vi "Receive - UDP (CommPort).vi"() -> ()   [LabVIEW 2020]
uses:
  <instrlib>/AIM GmbH/_AIM 664/_controls/comm_verification_rx.ctl
  <instrlib>/AIM GmbH/_AIM 664/_controls/comm_udp_rx.ctl
  <instrlib>/AIM GmbH/_AIM 664/_polimorphicInstances/session/CreateSession(Rx-VL-Oriented).vi
  <instrlib>/AIM GmbH/_AIM 664/bsp/AFDX_Receive/Create Rx VL.vi
  <instrlib>/AIM GmbH/_AIM 664/_polimorphicInstances/udpPort/CreateUdpPort(RX-CommPort).vi
  <instrlib>/AIM GmbH/_AIM 664/_polimorphicInstances/control/Start (Rx).vi
  <instrlib>/AIM GmbH/_AIM 664/_polimorphicInstances/control/Stop (Rx).vi
  <instrlib>/AIM GmbH/_AIM 664/_polimorphicInstances/session/CleanupSession (Port).vi
  <instrlib>/AIM GmbH/_AIM 664/AIM664LV.lvlib
panel:
  out "Curent Irig Time":T1
  in  "CommPort Config":T2={"PortType"=enum."FDX_UDP_SAMPLING", "SubVIId"=1, "domainID"=1, "sideID"=1, "locationID"=1, "partitionID"=1, "UdpSrcPort"=12345, "UdpDstPort"=12346, "UdpNumBufMessages"=0, "UdpMaxMessageSize"=1000, "UdpSamplingRate"=0} {"partitionID" format="%.0b"}
  out "BytesRead":u32
  out "Data":u8[](array[numeric])=[1, 2, 3, 4, 0, 0, 0, 0, 0, 0, 0, 0, 0, 0, 0, 0, 0, 0, 0, 0, 0, 0, 0, 0, 0, 0, 0, 0, 0, 0, 0, 0, 0, 0, 0, 0, 0, 0, 0, 0, 0, 0, 0, 0, 0, 0, 0, 0, 0, 0, 0, 0, 0, 0, 0, 0, 0, 0, 0, 0, 0, 0, 0, 0, 0, 0, 0, 0, 0, 0, 0, 0, 0, 0, 0, 0, 0, 0, 0, 0, 0, 0, 0, 0, 0, 0, 0, 0, 0, 0, 0, 0, 0, 0, 0, 0, 0, 0, 0, 0] format="%.0x"
  in  "Messages to Read (1)":u32=1
  in  "VL Config":T3={"VlId"=60, "VLRange"=1, "VerificationMode"=0, "Bag"=0, "Jitter"=0, "MaxFrameLength"=0, "MaxSkew"=0, "VLBufSize"=32768, "FilterMode"=0, "FilterPosition"=0, "Padding"=0, "FilterMask"=0, "FilterData"=0, "MinFrameLength"=0} {"FilterMode" items=["FDX_RX_VL_FLT_DIS", "FDX_RX_VL_FLT_ENA ", "FDX_RX_VL_FLT_ENA_INV"]; "MaxFrameLength" format="%.0x"; "VerificationMode" items=["FDX_RX_VL_CHECK_ENA_DEFAULT"=65535, "FDX_RX_VL_CHECK_REDMAM"=16, "DX_RX_VL_CHECK_TRAFIC"=8, "FDX_RX_VL_CHECK_FRAMESIZE"=4, "FDX_RX_VL_CHECK_SNINTEG"=2, "FDX_RX_VL_CHECK_INVPAC"=1, "FDX_RX_VL_CHECK_DISA"=0]}
  out "PortInitOut":T4 {"PortConfig" items=["FDX_SINGLE", "FDX_REDUNDANT"]}
  in  "port":u32=1
  in  "board":u32
  in  "Period mS":u32=200
  out "error out":errorcluster
  in  "stop":bool
  out "current time":timestamp
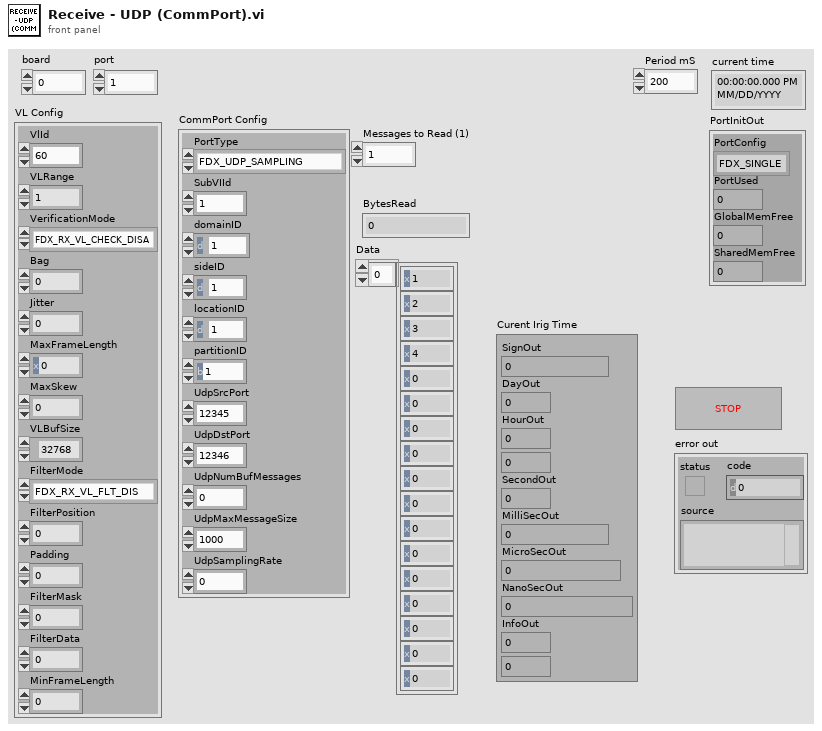
[diagram p1: front panel]
types:
  T1 = cluster{"SignOut":i32, "DayOut":u32, "HourOut":u32, "MinOut":u32, "SecondOut":u32, "MilliSecOut":u32, "MicroSecOut":u32, "NanoSecOut":u32, "InfoOut":u32, "Mode":u32}
  T2 = typedef "AIM664LV.lvlib/comm_udp_rx.ctl" = cluster{"PortType":enum16{"FDX_UDP_SAMPLING", "FDX_UDP_QUEUING"}, "SubVIId":u32, "domainID":u8, "sideID":u8, "locationID":u8, "partitionID":u8, "UdpSrcPort":u16, "UdpDstPort":u16, "UdpNumBufMessages":u32, "UdpMaxMessageSize":u32, "UdpSamplingRate":u32}
  T3 = typedef "AIM664LV.lvlib/comm_verification_rx.ctl" = cluster{"VlId":u16, "VLRange":u32, "VerificationMode":u32, "Bag":u32, "Jitter":u32, "MaxFrameLength":u32, "MaxSkew":u32, "VLBufSize":u32, "FilterMode":u32, "FilterPosition":u32, "Padding":u32, "FilterMask":u32, "FilterData":u32, "MinFrameLength":u32}
  T4 = cluster{"PortConfig":u32, "PortUsed":u32, "GlobalMemFree":u32, "SharedMemFree":u32}
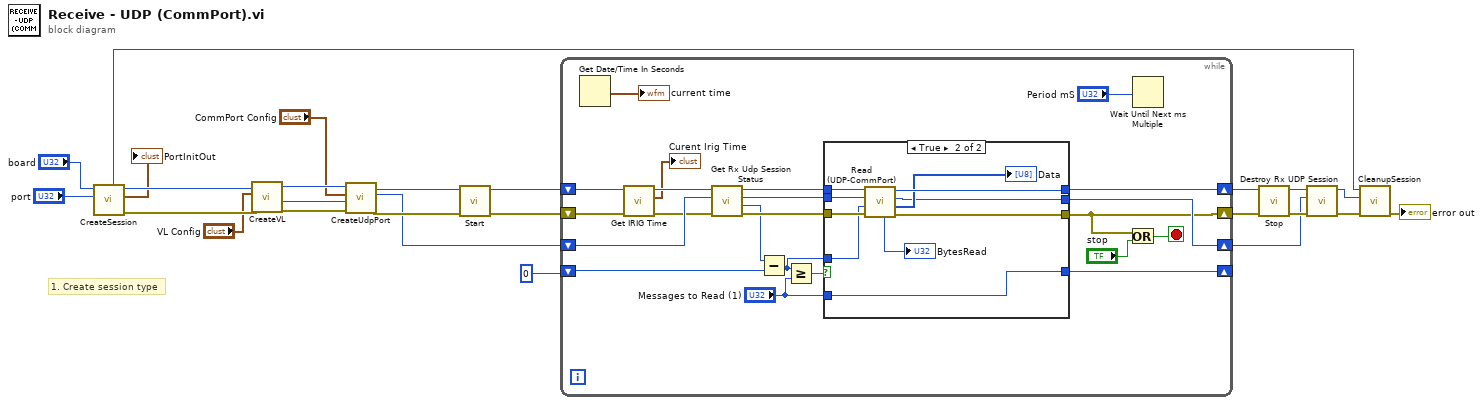
[diagram p0: block diagram]
diagram:
  # "1. Create session type"
  n1 = call-poly <instrlib>:"CreateSession.vi"("port"="port", "board"="board") -> ("error out"=w24:errorcluster, "PortInitOut"=→"PortInitOut":T4, "InstrumentHandle_port out"=w25:u32, "InstrumentHandle_board out"=w5:u32)  [unwired: 4 in, 2 out]
  n2 = call-poly <instrlib>:"CreateVL.vi"("error in (no error)"=w24, "VL Config"="VL Config", "InstrumentHandle_port in"=w25) -> ("error out"=w22:errorcluster, "VlId"=w8:u16, "InstrumentHandle_port out"=w23:u32)  [unwired: 6 in]
  n3 = call-poly <instrlib>:"CreateUdpPort.vi"("error in (no error)"=w22, "VlId"=w8, "CommPort Config"="CommPort Config", "port handle in"=w23) -> ("error out"=w20:errorcluster, "commPort handle out"=w17:u32, "port handle out"=w21:u32)  [unwired: 4 in, 1 out]
  n4 = call-poly <instrlib>:"Start.vi"("error in (no error)"=w20, "InstrumentHandle_port in"=w21) -> ("error out"=w2:errorcluster, "InstrumentHandle_port out"=w19:u32)  [unwired: 8 in]
  n5 = while {
    shift-right: [w39] -> w18
    shift-left: w19 -> [w34]
    shift-right: [w35] -> w3
    shift-left: w17 -> [w38]
    shift-right: [w40] -> _
    shift-left: u32 0 ("MsgCount") -> [w46]
    shift-right: [w26] -> w1
    shift-left: w2 -> [w29]
    stop <- w28 stop-if-true
    n6 = Get Date/Time In Seconds() -> (seconds since 1Jan1904=→"current time":timestamp)
    n7 = call <instrlib>:"Get IRIG Time.vi"("error in (no error)"=w29, "InstrumentHandle_board in"=w34) -> ("error out"=w33:errorcluster, "Curent Irig Time"=→"Curent Irig Time":T1, "InstrumentHandle_board out"=w32:u32)  [unwired: 7 in]
    n8 = call <instrlib>:"Get Rx Udp Session Status.vi"("error in (no error)"=w33, "UdpHandle in"=w38, "InstrumentHandle_port in"=w32) -> ("error out"=w45:errorcluster, "MsgCount"=w36:u32, "UdpHandle out"=w37:u32, "InstrumentHandle_port out"=w44:u32)  [unwired: 4 in, 1 out]
    n9 = Subtract(x=w36, y=w46) -> (x-y=w41:u32)
    n10 = Greater Or Equal?(x=w41, y="Messages to Read (1)") -> (x >= y?=w43:bool)
    n11 = case shown="True" w43 {
      tunnel: w45 -> [w49 w59]
      tunnel: w44 -> [w51 w60]
      tunnel: "Messages to Read (1)" -> [_ w61]
      tunnel: [w51 w58] -> w39
      tunnel: w41 -> [w50 w54]
      tunnel: [w50 w61] -> w40
      tunnel: [w49 w57] -> w26
      tunnel: w37 -> [w48 w55]
      tunnel: [w48 w52] -> w35
      frame False {
      }
      frame True {
        n12 = call <instrlib>:"Read (UDP-CommPort).vi"("error in (no error)"=w59, "MsgCount(1)"=w54, "UdpHandle in"=w55, "InstrumentHandle_port in"=w60) -> ("error out"=w57:errorcluster, "Data"=→"Data":u8[], "UdpHandle out"=w52:u32, "InstrumentHandle_port out"=w58:u32, "MsgRead"=→"BytesRead":u32)  [unwired: 3 in]
      }
    }
    n13 = Or(x=w26, y="stop") -> (x .or. y?=w28:bool)
    n14 = Wait Until Next ms Multiple(millisecond multiple="Period mS") -> ()  [unwired: 1 out]
  }
  n15 = call-poly <instrlib>:"Stop.vi"("error in (no error)"=w1, "InstrumentHandle_port in"=w18) -> ("error out"=w16:errorcluster, "InstrumentHandle_port out"=w4:u32)  [unwired: 8 in]
  n16 = call <instrlib>:"Destroy Rx UDP Session.vi"("error in (no error)"=w16, "UdpHandle in"=w3, "InstrumentHandle_port in"=w4) -> ("error out"=w15:errorcluster, "InstrumentHandle_port out"=w6:u32)  [unwired: 7 in]
  n17 = call-poly <instrlib>:"CleanupSession.vi"("error in (no error)"=w15, "InstrumentHandle_port in"=w6, "InstrumentHandle_board in"=w5) -> ("error out"=→"error out":errorcluster)  [unwired: 8 in]
